vi "Debug from Host.vi"() -> ()   [LabVIEW 2020]
panel:
  out "error out":errorcluster
  out "DebugString":string
  in  "stop":bool
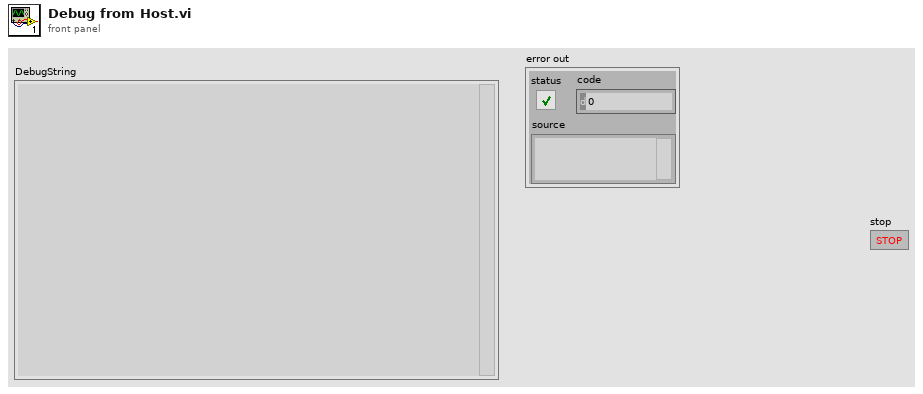
[diagram p1: front panel]
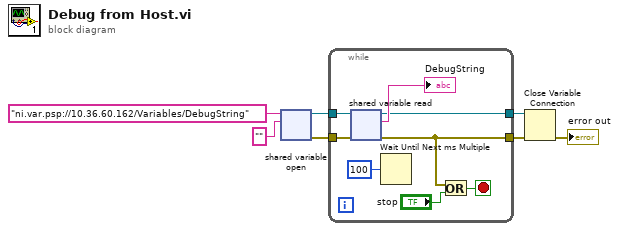
[diagram p0: block diagram]
diagram:
  n1 = shared-variable-open("ni.var.psp://10.36.60.162/Variables/DebugString" ("string"), "") -> (w5:refnum<k21>, w4:errorcluster)  [unwired: 2 in]
  n2 = while {
    tunnel: w4 -> [w13]
    tunnel: w5 -> [w14]
    tunnel: [w11] -> w3
    tunnel: [w8] -> w2
    stop <- w10 stop-if-true
    n3 = shared-variable-read(w14, w13) -> (w11:refnum<k21>, w8:errorcluster, →"DebugString":string)  [unwired: 1 out]
    n4 = Wait Until Next ms Multiple(millisecond multiple=u32 100) -> ()  [unwired: 1 out]
    n5 = Or(x=w8, y="stop") -> (x .or. y?=w10:bool)
  }
  n6 = Close Variable Connection(8:w2, 11:w3) -> (0:→"error out":errorcluster)
